vi "cyclical_counter_clk.vi"(1 "clk":bool, 2 "Mod":u16) -> (0 "Count":u16)   [LabVIEW 2018]
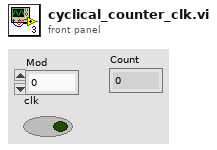
[diagram p1: front panel]
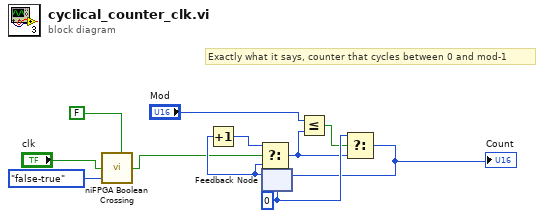
[diagram p0: block diagram]
diagram:
  w5 = u16 0
  # "Exactly what it says, counter that cycles between 0 and mod-1"
  n1 = call <vilib>:"niFPGA Boolean Crossing.vi"("input"="clk", "direction"=enum8{"either", "false-true", "true-false"}."false-true", "initialize"=FALSE) -> ("crossing"=w7:bool)  [unwired: 6 in]
  n2 = feedback #1(w5) -> (w10:u16)
  n3 = Increment(x=w10) -> (x+1=w11:u16)
  n4 = Select(t=w11, s=w7, f=w10) -> (s? t:f=w2:u16)
  n5 = Less Or Equal?(x="Mod", y=w2) -> (x <= y?=w4:bool)
  n6 = Select(t=w5, s=w4, f=w2) -> (s? t:f=w1:u16)
  "Count" <- w1
  n7 = feedback-in #1(w1) -> ()
